vi "Bulk Add Helper.vi"(10 "Add VI In":refnum<vi>, 11 "Node Ptr":T1 format="%.0x") -> ()   [LabVIEW 2015, in "Modbus Master System Explorer.lvlib"]
uses:
  Modbus Master System Explorer.lvlib
  <vilib>/NI Veristand/Custom Device API/Custom Device Item Ref.ctl
  Modbus Type.ctl
  Shared/Controls/Data Model/Mapping.ctl
  Shared/Controls/Data Model/DataType.ctl
  <vilib>/NI VeriStand/Custom Device API/Custom Device API.lvlib
  Shared/Modbus Master Shared.lvlib
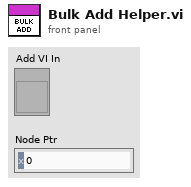
[diagram p1: front panel]
types:
  T1 = typedef "Custom Device API.lvlib/Custom Device Item Ref.ctl" = u64
  T2 = typedef "Modbus Master Shared.lvlib/Modbus Type.ctl" = enum16{"Coil", "Discrete Input", "Holding Register", "Input Register"}
  T3 = typedef "Modbus Master Shared.lvlib/DataType.ctl" = enum16{"Double", "Single", "I64", "I32", "I16", "I8", "U64", "U32", "U16", "U8", "Boolean"}
  T4 = typedef "Modbus Master Shared.lvlib/Mapping.ctl" = cluster{"DataType":T3, "Starting Address":u16, "Sub-Index (Bool)":u16, "VS Reference":T1}
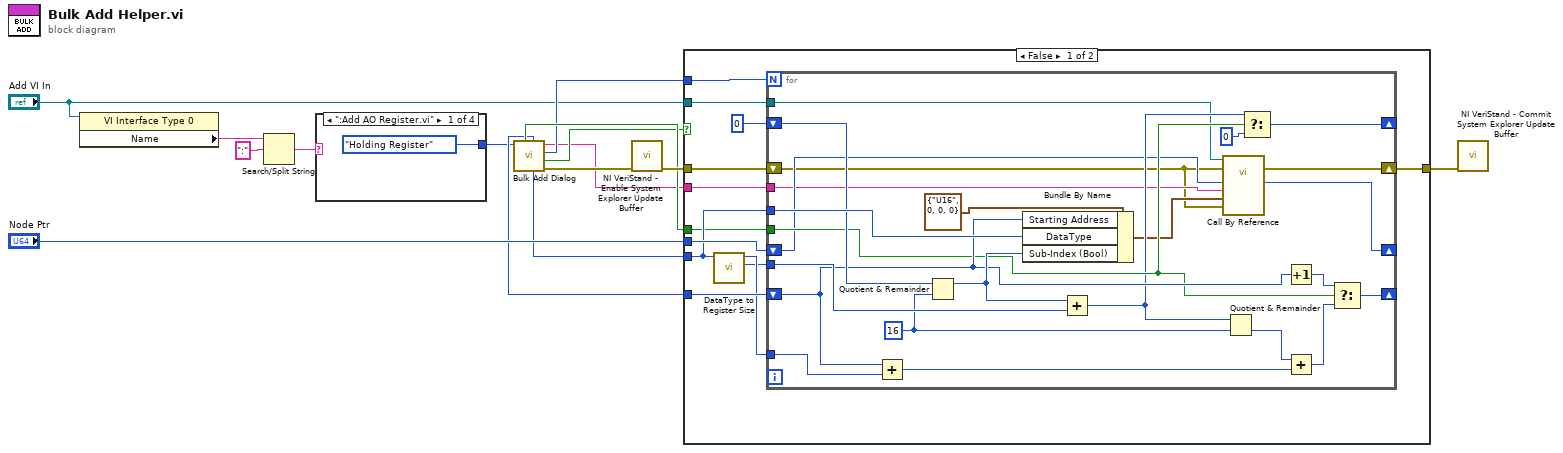
[diagram p0: block diagram]
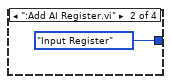
[diagram p2: hidden frame]
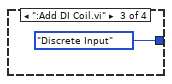
[diagram p3: hidden frame]
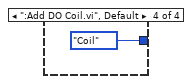
[diagram p4: hidden frame]
diagram:
  n1 = property class="VI Interface Type 0"(reference="Add VI In") -> ("Name"=w3:string)  [unwired: 1 in, 2 out]
  n2 = Search/Split String(string=w3, search string/char (-)=":") -> (match + rest of string=w2:string)  [unwired: 1 in, 2 out]
  n3 = case shown="\":Add AO Register.vi\"" w2 {
    tunnel: [Modbus_Type."Holding Register" ("Type") Modbus_Type."Input Register" ("Type") Modbus_Type."Discrete Input" ("Type") Modbus_Type."Coil" ("Type")] -> w1
    frame ":Add AO Register.vi" {
    }
    frame ":Add AI Register.vi" {
    }
    frame ":Add DI Coil.vi" {
    }
    frame ":Add DO Coil.vi", Default {
    }
  }
  n4 = call "Bulk Add Dialog.vi"("Type"=w1) -> ("error out"=w14:errorcluster, "Cancelled?"=w9:bool, "Quantity Out"=w8:u16, "Root Name Out"=w7:string, "DataType Out"=w10:T3, "Starting Address Out"=w6:u16, "Pack Values? Out"=w12:bool)  [unwired: 4 in]
  n5 = call <vilib>:"NI VeriStand - Enable System Explorer Update Buffer.vi"("error in (no error)"=w14) -> ("error out"=w15:errorcluster)  [unwired: 10 in]
  n6 = case shown="False" w9 {
    tunnel: "Node Ptr" -> [w24 _]
    tunnel: w8 -> [w31 _]
    tunnel: w15 -> [w25 w56]
    tunnel: w7 -> [w30 _]
    tunnel: w6 -> [w29 _]
    tunnel: w10 -> [w23 _]
    tunnel: w12 -> [w22 _]
    tunnel: [w21 w56] -> w13
    tunnel: "Add VI In" -> [w20 _]
    frame False {
      n7 = call "DataType to Register Size.vi"("DataType"=w23) -> ("bits"=w26:i32, "bytes"=w28:i32)  [unwired: 9 in]
      n8 = for {
        N: w31 -> [_]
        shift-right: [w32] -> _
        shift-left: w24 -> [w36]
        shift-right: [w37] -> w21
        shift-left: w25 -> [w33]
        tunnel: w30 -> [w35]
        shift-right: [w45] -> _
        shift-left: w29 -> [w46]
        tunnel: w23 -> [w54]
        tunnel: w28 -> [w53]
        shift-right: [w42] -> _
        shift-left: 0 ("Sub-Index (Bool)") -> [w51]
        tunnel: w26 -> [w52]
        tunnel: w22 -> [w44]
        tunnel: w20 -> [w38]
        w48 = 16 ("y")
        n9 = Add(x=w46, y=w53) -> (x+y=w49:i32)
        n10 = Quotient & Remainder(x=w51, y=w48) -> (x-y*floor(x/y)=w50:i32)  [unwired: 1 out]
        n11 = Bundle By Name(cluster=T4 {"DataType"=enum."U16", "Starting Address"=0, "Sub-Index (Bool)"=0, "VS Reference"=0} ("Mapping"), "Starting Address"=w46, "DataType"=w54, "Sub-Index (Bool)"=w50) -> (w34:T4)
        n12 = Add(x=w50, y=w52) -> (x+y=w43:i32)
        n13 = call-by-ref "?"(reference=w38, error in=w33, 8:"error in (no error)"=w33, "Mapping"=w34, "Label"=w35, "Node Ref In"=w36) -> (error out=w37:errorcluster, "Node Ref out"=w32:T1)  [unwired: 5 in, 3 out]
        n14 = Quotient & Remainder(x=w43, y=w48) -> (floor(x/y)=w47:i32)  [unwired: 1 out]
        n15 = Select(t=w43, s=w44, f=0 ("t")) -> (s? t:f=w42:i32)
        n16 = Increment(x=w46) -> (x+1=w39:i32)
        n17 = Add(x=w47, y=w49) -> (x+y=w40:i32)
        n18 = Select(t=w39, s=w44, f=w40) -> (s? t:f=w45:i32)
      }
    }
    frame True {
    }
  }
  n19 = call <vilib>:"NI VeriStand - Commit System Explorer Update Buffer.vi"("error in (no error)"=w13) -> ()  [unwired: 10 in, 1 out]
